vi "bats.parser.vi"(8 "FIFO In":refnum<k21>="TS-OrderBook.Command", 9 "reset":bool, 10 "data_valid":bool, 11 "data":u8) -> (3 "Ready for Input":bool)   [LabVIEW 2020]
uses:
  bats.parser.state.data.ctl
  bats.parser.state.command.ctl
  orderbook/orderbook.command.data.ctl
  orderbook/orderbook.command.type.ctl
  <vilib>/rvi/DataTransferAndStorage/Container/Common/niFpgaContainerExecOnDevCompGetState.vi
  <vilib>/rvi/Emulation/niFpgaEmulationIsFPGAContextNoSignature.vi
  <vilib>/rvi/Emulation/niFpgaSctlEmulationGetInTimedLoop.vi
  <vilib>/rvi/errors/niFpgaSetErrorForExecOnDevCompSimple.vi
  <vilib>/rvi/eio/common/nirviEmuReportErrorAndStop.vi
  <vilib>/rvi/DataTransferAndStorage/Container/Common/niFpgaContainerGetUniqueNameForEmu.vi
  <vilib>/rvi/FIFO/Fifo_Resource/nirvififoEmulationSetSize.vi
  <vilib>/rvi/FIFO/Fifo_Resource/nirviFifoEmulationQueueMgr.vi
  <instcachedir>/0/nirviFifoEmulationQueueMgr_E5CAEC123FF24DC58D834DCA3CDAA9B5.lvgen/nirviFifoEmulationQueueMgr_E5CAEC123FF24DC58D834DCA3CDAA9B5_016.vi
  <vilib>/rvi/FIFO/Fifo_Resource/nirvififoEmulationDetermineInputValidOut.vi
  <vilib>/rvi/FIFO/Fifo_Resource/nirvififoEmulationCreateLock.vi
  <vilib>/rvi/Emulation/niFpgaProcessEmulError.vi
  <vilib>/rvi/FIFO/Fifo_Resource/nirvififoEmulationObtainLock.vi
  <vilib>/rvi/FIFO/Fifo_Resource/nirvififoEmulationReleaseLock.vi
  <vilib>/rvi/occurrence/nirviWaitOnOccurrenceBase.vi
  <vilib>/rvi/errors/nirviReportUnexpectedCaseInternalError.vi
  <vilib>/rvi/errors/nirviReportUnexpectedCaseInternalError (U32).vi
  <vilib>/Utility/error.llb/Clear Errors.vi
  <vilib>/rvi/interface/RandomDataEmulation/niFpgaRandomDataHandleErrors.vi
  <vilib>/rvi/DataTransferAndStorage/Container/XNode/niFpgaContainer.xnode
  <vilib>/rvi/FIFO/Fifo_Resource/niFpgaFifoEmulationRefIn.vi
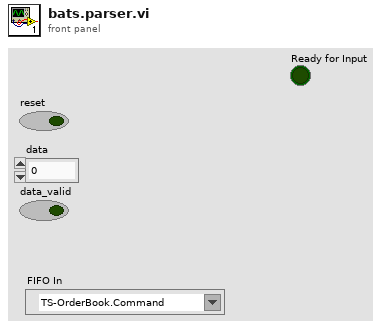
[diagram p1: front panel]
types:
  T1 = typedef "bats.parser.state.command.ctl" = enum16{"Send.Command", "Reset", "No.Op", "Read.Sequenced.Unit.Header", "Read.Msg.Type.and.Length", "Read.Time", "Read.Add.Order", "Read.Order.Executed", "Read.Reduce.Size", "Read.Modify.Order", "Read.Delete.Order"}
  T2 = typedef "orderbook.command.data.ctl" = cluster{"OrderBook Command":T3, "Side (U8)":u8, "Order Id (U64)":u64, "Quantity (U32)":u32, "Symbol (U64)":u64, "Price (U64)":u64, "Executed Quantity (U32)":u32, "Cancelled Quantity (U32)":u32}
  T3 = typedef "orderbook.command.type.ctl" = enum16{"AddOrder", "OrderExecuted", "ReduceSize", "ModifyOrder", "DeleteOrder"}
  T4 = typedef "bats.parser.state.data.ctl" = cluster{"BATS.Parser.States":T1, "Hdr Length (U16)":u16, "MessageLength (U8)":u8, "MessageType (U8)":u8, "Time (U32)":u32, "Total Counter (U16)":u16, "Message Counter (U8)":u8}
  T5 = cluster{"BATS.Parser.States":enum16{"Read.Sequenced.Unit.Header", "Read.Msg.Type.and.Length", "Read.Time", "Read.Add.Order", "Read.Order.Executed", "Read.Reduce.Size", "Read.Modify.Order", "Read.Delete.Order"}, "Hdr Length (U16)":u16, "MessageLength (U8)":u8, "MessageType (U8)":u8, "Time (U32)":u32, "Total Counter (U16)":u16, "Message Counter (U8)":u8}
  T6 = cluster{"OrderBook Command":enum16{"AddOrder", "OrderExecuted", "ReduceSize", "ModifyOrder", "DeleteOrder"}, "Side (U8)":u8, "Order Id (U64)":u64, "Quantity (U32)":u32, "Symbol (U64)":u64, "Price (U64)":u64, "Executed Quantity (U32)":u32, "Cancelled Quantity (U32)":u32}
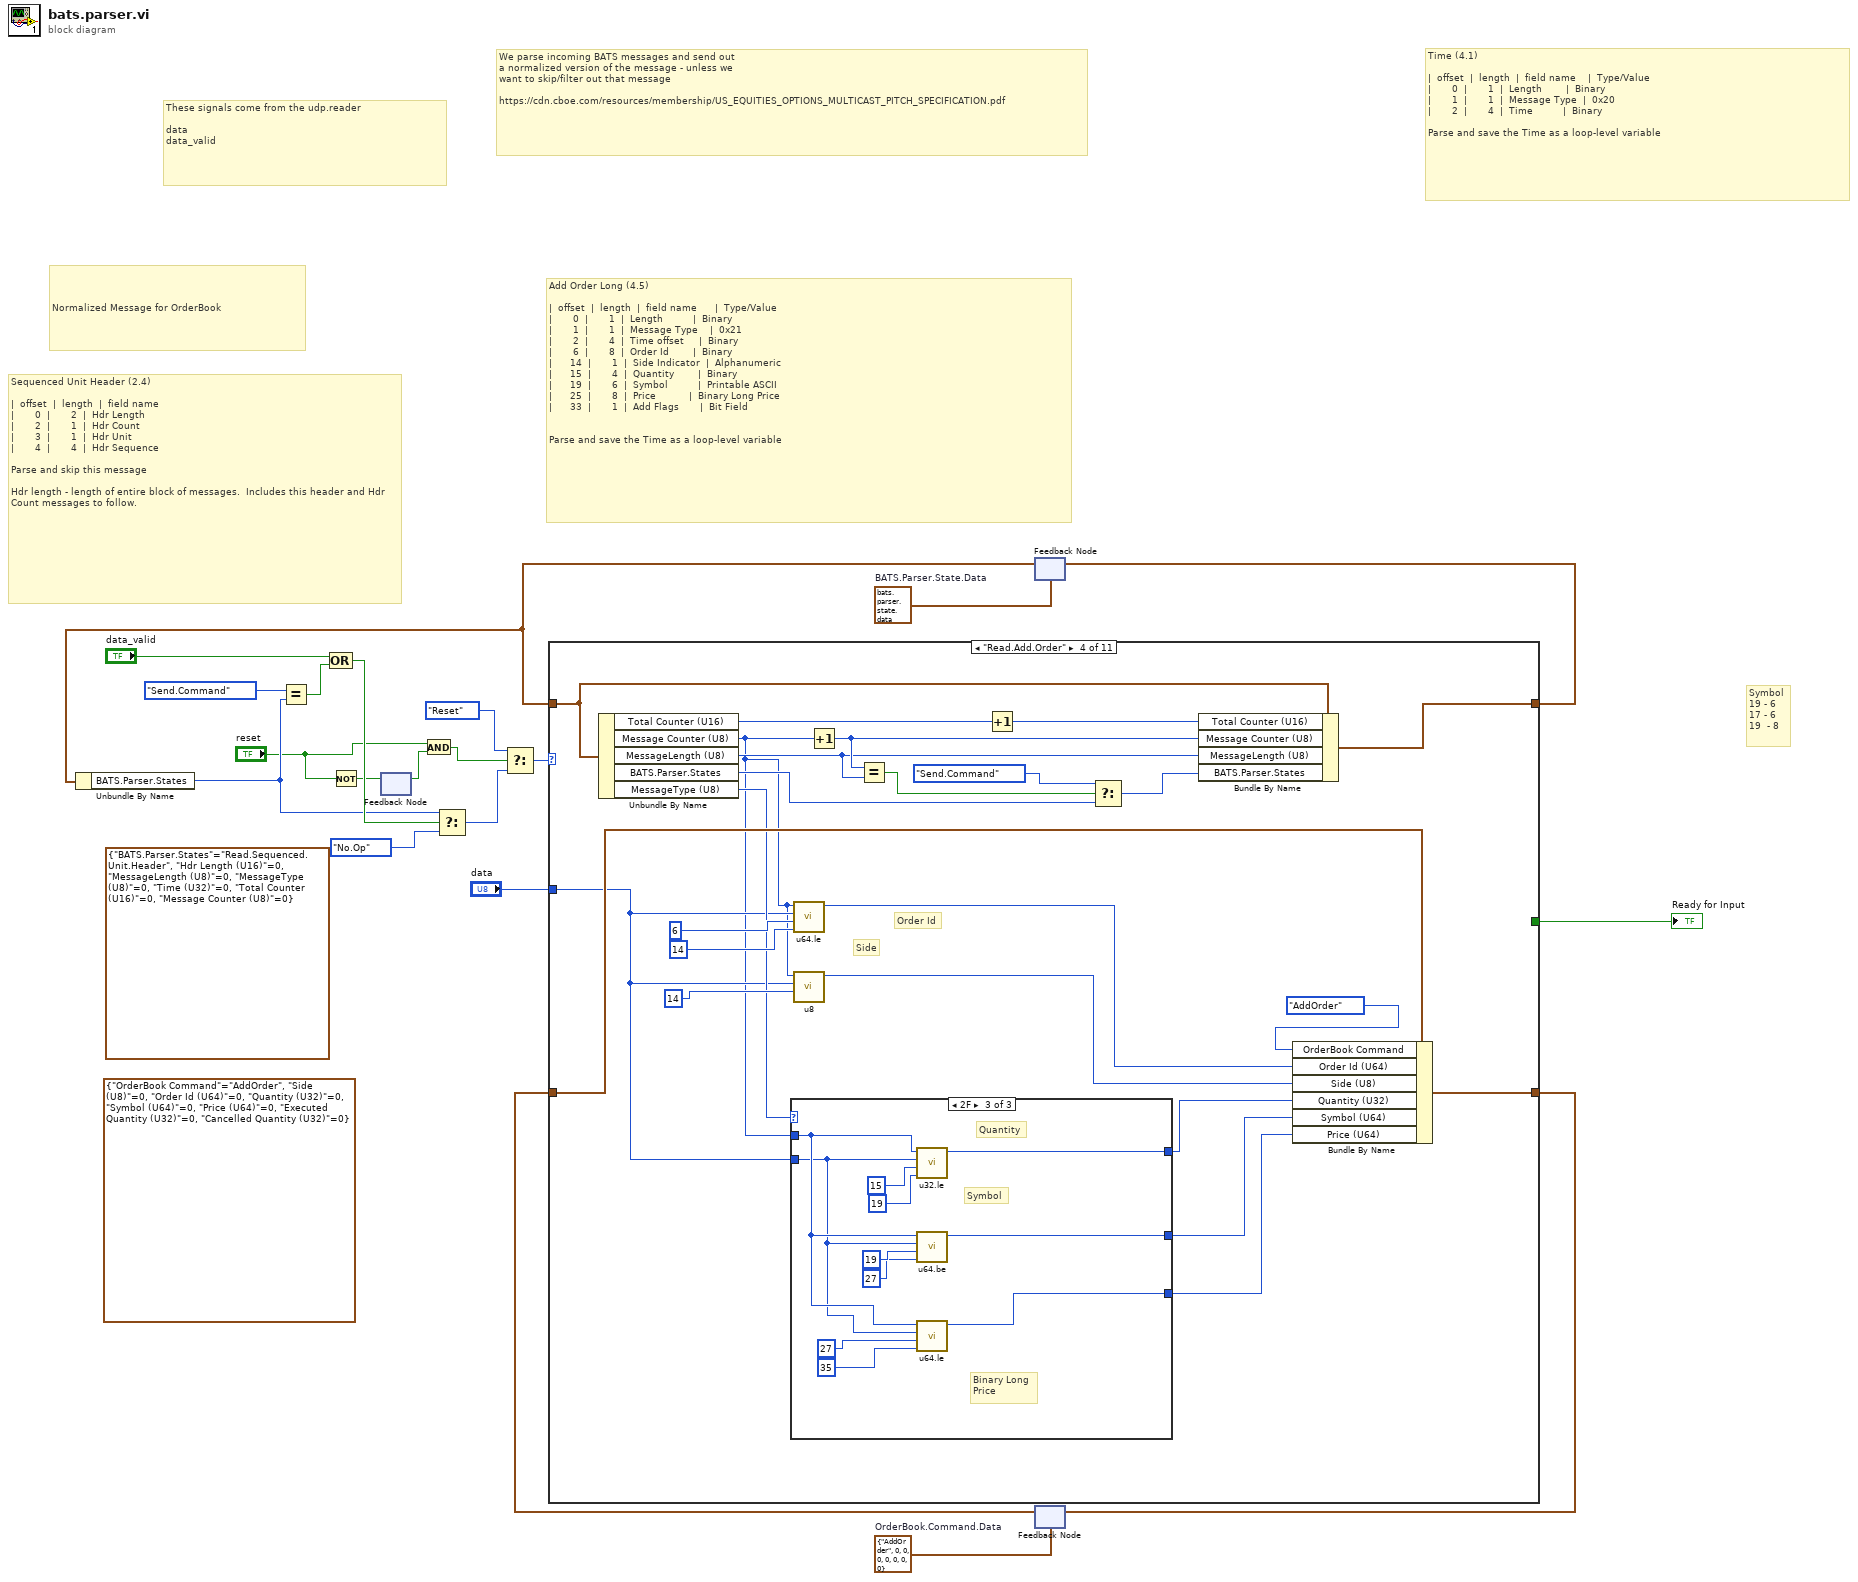
[diagram p0: block diagram]
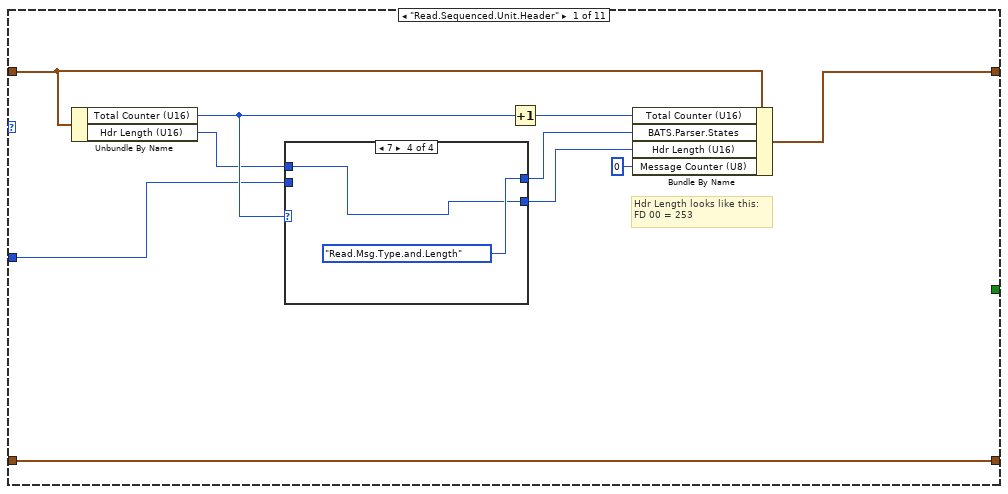
[diagram p2: hidden frame]
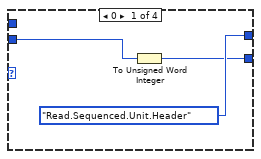
[diagram p3: hidden frame]
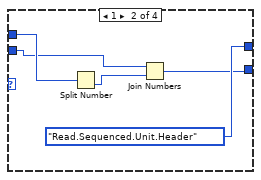
[diagram p4: hidden frame]
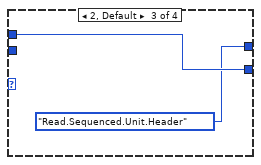
[diagram p5: hidden frame]
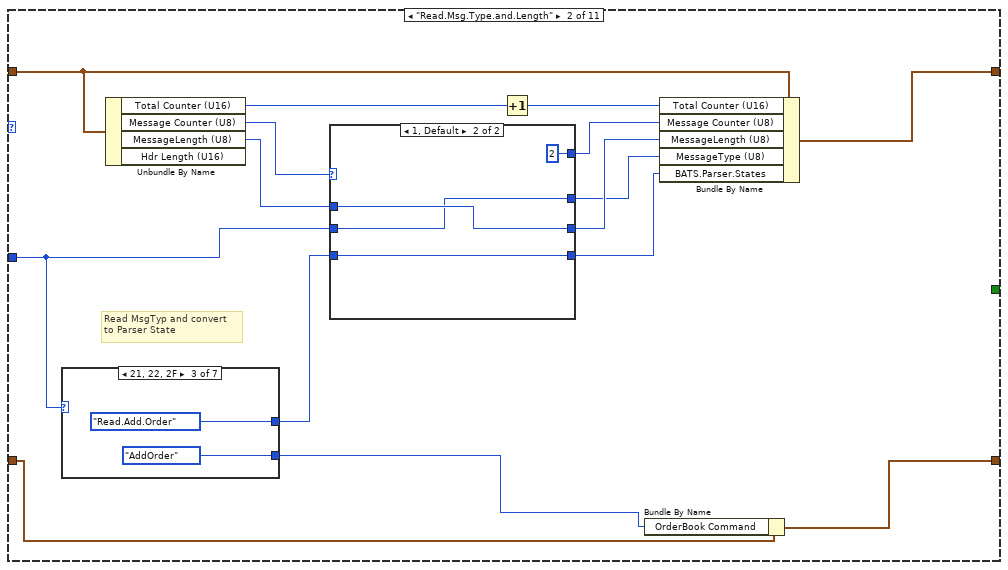
[diagram p6: hidden frame]
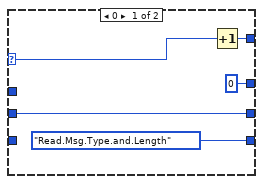
[diagram p7: hidden frame]
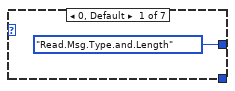
[diagram p8: hidden frame]
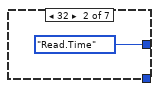
[diagram p9: hidden frame]
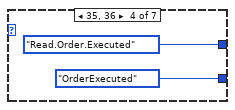
[diagram p10: hidden frame]
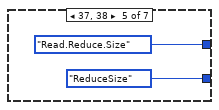
[diagram p11: hidden frame]
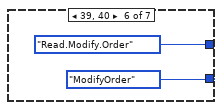
[diagram p12: hidden frame]
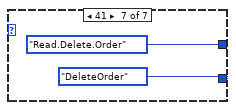
[diagram p13: hidden frame]
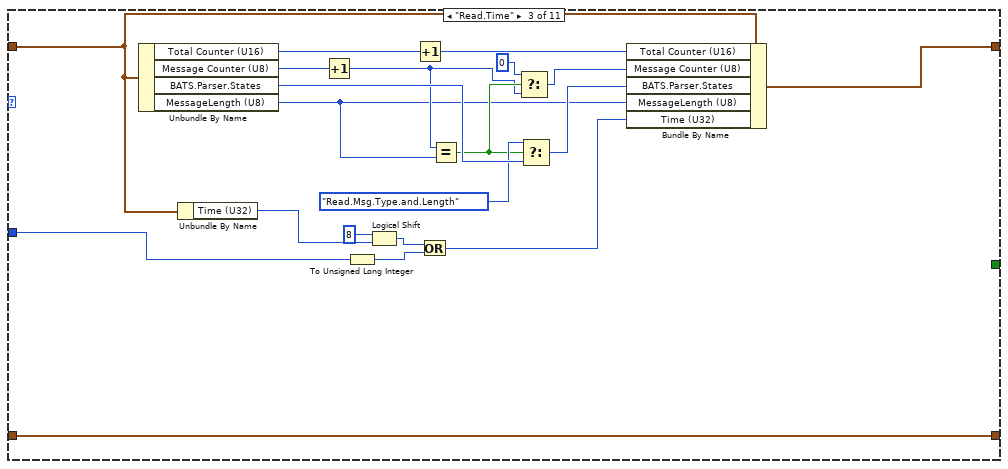
[diagram p14: hidden frame]
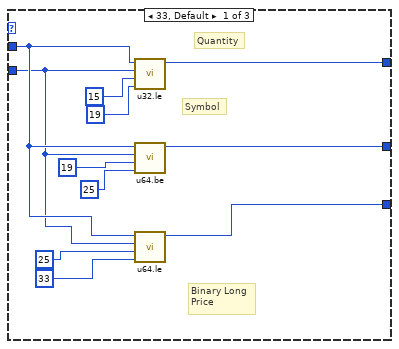
[diagram p15: hidden frame]
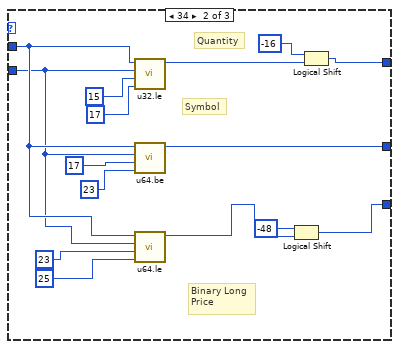
[diagram p16: hidden frame]
diagram:
  w17 = T2 {"OrderBook Command"=enum."AddOrder", "Side (U8)"=0, "Order Id (U64)"=0, "Quantity (U32)"=0, "Symbol (U64)"=0, "Price (U64)"=0, "Executed Quantity (U32)"=0, "Cancelled Quantity (U32)"=0}  # OrderBook.Command.Data
  w18 = T4 {"BATS.Parser.States"=enum."Read.Sequenced.Unit.Header", "Hdr Length (U16)"=0, "MessageLength (U8)"=0, "MessageType (U8)"=0, "Time (U32)"=0, "Total Counter (U16)"=0, "Message Counter (U8)"=0}  # BATS.Parser.State.Data
  (unwired) T5 {"BATS.Parser.States"=enum."Read.Sequenced.Unit.Header", "Hdr Length (U16)"=0, "MessageLength (U8)"=0, "MessageType (U8)"=0, "Time (U32)"=0, "Total Counter (U16)"=0, "Message Counter (U8)"=0}
  (unwired) T6 {"OrderBook Command"=enum."AddOrder", "Side (U8)"=0, "Order Id (U64)"=0, "Quantity (U32)"=0, "Symbol (U64)"=0, "Price (U64)"=0, "Executed Quantity (U32)"=0, "Cancelled Quantity (U32)"=0}
  # "Symbol\n19 - 6\n17 - 6\n19  - 8"
  # "Sequenced Unit Header (2.4)\n\n|  offset  |  length  |  field name\n|       0  |       2  |  Hdr Length\n|       2  |       1  |  Hdr Count\n|       3  |       1  |  Hdr Unit\n|       4  |       4  |  Hdr Sequence\n\nParse and skip this message\n\nHdr length - length of entire block of messages.  Includes this header and Hdr Count messages to follow."
  # "Normalized Message for OrderBook"
  # "Add Order Long (4.5)\n\n|  offset  |  length  |  field name      |  Type/Value\n|       0  |       1  |  Length          |  Binary\n|       1  |       1  |  Message Type    |  0x21\n|       2  |       4  |  Time offset     |  Binary\n|       6  |       8  |  Order Id        |  Binary\n|      14  |       1  |  Side Indicator  |  Alphanumeric\n|      15  |       4  |  Quantity        |  Binary\n|      19  |       6  |  Symbol          |  Printable ASCII\n|      25  |       8  |  Price           |  Binary Long Price\n|      33  |       1  |  Add Flags       |  Bit Field\n\n\nParse and save the Time as a loop-level variable"
  # "Time (4.1)\n\n|  offset  |  length  |  field name    |  Type/Value\n|       0  |       1  |  Length        |  Binary\n|       1  |       1  |  Message Type  |  0x20\n|       2  |       4  |  Time          |  Binary\n\nParse and save the Time as a loop-level variable"
  # "We parse incoming BATS messages and send out\na normalized version of the message - unless we\nwant to skip/filter out that message\n\nhttps://cdn.cboe.com/resources/membership/US_EQUITIES_OPTIONS_MULTICAST_PITCH_SPECIFICATION.pdf"
  # "These signals come from the udp.reader\n\ndata\ndata_valid"
  n1 = Not(x="reset") -> (.not. x?=w2:bool)
  n2 = feedback-in #1(w2) -> ()
  n3 = feedback #1() -> (w3:bool)  [unwired: 1 in]
  n4 = And(x="reset", y=w3) -> (x .and. y?=w4:bool)
  n5 = feedback #2(w18) -> (w14:T4)
  n6 = Unbundle By Name(w14) -> ("BATS.Parser.States"=w6:T1)
  n7 = Equal?(x=bats.parser.state.command."Send.Command" ("BATS.Parser.States"), y=w6) -> (x = y?=w7:bool)
  n8 = Compound Arithmetic op=OR("data_valid", w7) -> (w9:bool)
  n9 = Select(t=w6, s=w9, f=bats.parser.state.command."No.Op" ("BATS.Parser.States")) -> (s? t:f=w11:T1)
  n10 = Select(t=bats.parser.state.command."Reset" ("BATS.Parser.States"), s=w4, f=w11) -> (s? t:f=w12:T1)
  n11 = feedback #3(w17) -> (w20:T2)
  n12 = case shown="\"Read.Add.Order\"" w12 {
    tunnel: w14 -> [w27 w57 w90 w119 w161 w163 w165 w167 _ w190 w200]
    tunnel: [w25 w54 w84 w116 w162 w164 w166 w168 w174 w189 w194] -> w21
    tunnel: w20 -> [w25 w55 w84 w114 w162 w164 w166 w168 _ w189 w194]
    tunnel: [w30 w58 w98 w117 w161 w163 w165 w167 w186 w190 w199] -> w19
    tunnel: "data" -> [w23 w47 w80 w102 _ _ _ _ _ _ _]
    tunnel: [_ _ _ _ _ _ _ _ _ TRUE ("Ready for Input") w191] -> w1
    frame "Read.Sequenced.Unit.Header" {
      # "Hdr Length looks like this:\nFD 00 = 253"
      n13 = Unbundle By Name(w27) -> ("Total Counter (U16)"=w29:u16, "Hdr Length (U16)"=w28:u16)
      n14 = case shown="7" w29 {
        tunnel: w28 -> [_ w38 w41 w42]
        tunnel: w23 -> [w33 w37 _ _]
        tunnel: [w32 w35 w41 w42] -> w22
        tunnel: [bats.parser.state.command."Read.Sequenced.Unit.Header" ("BATS.Parser.States") bats.parser.state.command."Read.Sequenced.Unit.Header" ("BATS.Parser.States") bats.parser.state.command."Read.Sequenced.Unit.Header" ("BATS.Parser.States") bats.parser.state.command."Read.Msg.Type.and.Length" ("BATS.Parser.States")] -> w26
        frame 0 {
          n15 = To Unsigned Word Integer(number=w33) -> (unsigned 16bit integer=w32:u16)
        }
        frame 1 {
          n16 = Split Number(x=w38) -> (lo(x)=w36:u8)  [unwired: 1 out]
          n17 = Join Numbers(hi=w37, lo=w36) -> ((hi.lo)=w35:u16)
        }
        frame 2, Default {
        }
        frame 7 {
        }
      }
      n18 = Increment(x=w29) -> (x+1=w24:u16)
      n19 = Bundle By Name(cluster=w27, "Total Counter (U16)"=w24, "BATS.Parser.States"=w26, "Hdr Length (U16)"=w22, "Message Counter (U8)"=u8 0) -> (w30:T4)
    }
    frame "Read.Msg.Type.and.Length" {
      # "Read MsgTyp and convert\nto Parser State"
      n20 = case shown="21, 22, 2F" w47 {
        tunnel: [bats.parser.state.command."Read.Msg.Type.and.Length" ("BATS.Parser.States") bats.parser.state.command."Read.Time" ("BATS.Parser.States") bats.parser.state.command."Read.Add.Order" ("BATS.Parser.States") bats.parser.state.command."Read.Order.Executed" ("BATS.Parser.States") bats.parser.state.command."Read.Reduce.Size" ("BATS.Parser.States") bats.parser.state.command."Read.Modify.Order" ("BATS.Parser.States") bats.parser.state.command."Read.Delete.Order" ("BATS.Parser.States")] -> w49
        tunnel: [_ _ orderbook.command.type."AddOrder" ("OrderBook Command") orderbook.command.type."OrderExecuted" ("OrderBook Command") orderbook.command.type."ReduceSize" ("OrderBook Command") orderbook.command.type."ModifyOrder" ("OrderBook Command") orderbook.command.type."DeleteOrder" ("OrderBook Command")] -> w53
        frame 0, Default {
        }
        frame 32 {
        }
        frame 33, 34, 47 {
        }
        frame 35, 36 {
        }
        frame 37, 38 {
        }
        frame 39, 40 {
        }
        frame 41 {
        }
      }
      n21 = Unbundle By Name(w57) -> ("Total Counter (U16)"=w45:u16, "Message Counter (U8)"=w46:u8, "MessageLength (U8)"=w52:u8)  [unwired: 1 out]
      n22 = case shown="1, Default" w46 {
        selector: w46 -> [w60 _]
        tunnel: w52 -> [_ w67]
        tunnel: [w63 w67] -> w51
        tunnel: w47 -> [w63 w66]
        tunnel: [bats.parser.state.command."Read.Msg.Type.and.Length" ("BATS.Parser.States") w65] -> w50
        tunnel: w49 -> [_ w65]
        tunnel: [u8 0 ("data") w66] -> w48
        tunnel: [w59 u8 2] -> w44
        frame 0 {
          n23 = Increment(x=w60) -> (x+1=w59:u8)
        }
        frame 1, Default {
        }
      }
      n24 = Increment(x=w45) -> (x+1=w56:u16)
      n25 = Bundle By Name(cluster=w55, "OrderBook Command"=w53) -> (w54:T2)
      n26 = Bundle By Name(cluster=w57, "Total Counter (U16)"=w56, "Message Counter (U8)"=w44, "MessageLength (U8)"=w51, "MessageType (U8)"=w48, "BATS.Parser.States"=w50) -> (w58:T4)
    }
    frame "Read.Time" {
      n27 = Unbundle By Name(w90) -> ("Total Counter (U16)"=w99:u16, "Message Counter (U8)"=w81:u8, "BATS.Parser.States"=w96:T1, "MessageLength (U8)"=w82:u8)
      n28 = Unbundle By Name(w90) -> ("Time (U32)"=w89:u32)
      n29 = Increment(x=w81) -> (x+1=w83:u8)
      n30 = To Unsigned Long Integer(number=w80) -> (unsigned 32bit integer=w91:u32)
      n31 = Logical Shift(y=i16 8, x=w89) -> (x << y=w92:u32)
      n32 = Increment(x=w99) -> (x+1=w97:u16)
      n33 = Or(x=w92, y=w91) -> (x .or. y?=w88:u32)
      n34 = Equal?(x=w83, y=w82) -> (x = y?=w86:bool)
      n35 = Select(t=u8 0, s=w86, f=w83) -> (s? t:f=w87:u8)
      n36 = Select(t=bats.parser.state.command."Read.Msg.Type.and.Length", s=w86, f=w96) -> (s? t:f=w94:T1)
      n37 = Bundle By Name(cluster=w90, "Total Counter (U16)"=w97, "Message Counter (U8)"=w87, "BATS.Parser.States"=w94, "MessageLength (U8)"=w82, "Time (U32)"=w88) -> (w98:T4)
    }
    frame "Read.Add.Order" {
      # "Side"
      # "Order Id"
      n38 = Unbundle By Name(w119) -> ("Total Counter (U16)"=w123:u16, "Message Counter (U8)"=w100:u8, "MessageLength (U8)"=w115:u8, "BATS.Parser.States"=w113:T1, "MessageType (U8)"=w105:u8)
      n39 = case shown="2F" w105 {
        tunnel: w102 -> [w126 w143 w152]
        tunnel: w100 -> [w127 w144 w153]
        tunnel: [w132 w138 w158] -> w104
        tunnel: [w131 w147 w157] -> w103
        tunnel: [w128 w136 w154] -> w101
        frame 33, Default {
          # "Binary Long\nPrice"
          # "Symbol"
          # "Quantity"
          n40 = call "u32.le.vi"("end"=u8 19, "start"=u8 15, "Data"=w126, "Counter"=w127) -> ("Latched\nValue"=w132:u32)  [unwired: 7 in]
          n41 = call "u64.be.vi"("end"=u8 25, "start"=u8 19, "Data"=w126, "Counter"=w127) -> ("Latched\nValue"=w131:u64)  [unwired: 7 in]
          n42 = call "u64.le.vi"("end"=u8 33, "start"=u8 25, "Data"=w126, "Counter"=w127) -> ("Latched\nValue"=w128:u64)  [unwired: 7 in]
        }
        frame 34 {
          # "Binary Long\nPrice"
          # "Symbol"
          # "Quantity"
          n43 = call "u32.le.vi"("end"=u8 17, "start"=u8 15, "Data"=w143, "Counter"=w144) -> ("Latched\nValue"=w140:u32)  [unwired: 7 in]
          n44 = call "u64.be.vi"("end"=u8 23, "start"=u8 17, "Data"=w143, "Counter"=w144) -> ("Latched\nValue"=w147:u64)  [unwired: 7 in]
          n45 = call "u64.le.vi"("end"=u8 25, "start"=u8 23, "Data"=w143, "Counter"=w144) -> ("Latched\nValue"=w137:u64)  [unwired: 7 in]
          n46 = Logical Shift(y=i16 -48, x=w137) -> (x << y=w136:u64)
          n47 = Logical Shift(y=i16 -16, x=w140) -> (x << y=w138:u32)
        }
        frame 47 {
          # "Binary Long\nPrice"
          # "Symbol"
          # "Quantity"
          n48 = call "u32.le.vi"("end"=u8 19, "start"=u8 15, "Data"=w152, "Counter"=w153) -> ("Latched\nValue"=w158:u32)  [unwired: 7 in]
          n49 = call "u64.be.vi"("end"=u8 27, "start"=u8 19, "Data"=w152, "Counter"=w153) -> ("Latched\nValue"=w157:u64)  [unwired: 7 in]
          n50 = call "u64.le.vi"("end"=u8 35, "start"=u8 27, "Data"=w152, "Counter"=w153) -> ("Latched\nValue"=w154:u64)  [unwired: 7 in]
        }
      }
      n51 = call "u64.le.vi"("end"=u8 14, "start"=u8 6, "Data"=w102, "Counter"=w100) -> ("Latched\nValue"=w106:u64)  [unwired: 7 in]
      n52 = call "u8.vi"("idx"=u8 14 ("x"), "data in"=w102, "Message Counter (U8)"=w100) -> ("data out"=w107:u8)  [unwired: 8 in]
      n53 = Increment(x=w100) -> (x+1=w121:u8)
      n54 = Equal?(x=w121, y=w115) -> (x = y?=w120:bool)
      n55 = Increment(x=w123) -> (x+1=w122:u16)
      n56 = Select(t=bats.parser.state.command."Send.Command" ("BATS.Parser.States"), s=w120, f=w113) -> (s? t:f=w112:T1)
      n57 = Bundle By Name(cluster=w119, "Total Counter (U16)"=w122, "Message Counter (U8)"=w121, "MessageLength (U8)"=w115, "BATS.Parser.States"=w112) -> (w117:T4)
      n58 = Bundle By Name(cluster=w114, "OrderBook Command"=orderbook.command.type."AddOrder", "Order Id (U64)"=w106, "Side (U8)"=w107, "Quantity (U32)"=w104, "Symbol (U64)"=w103, "Price (U64)"=w101) -> (w116:T2)
    }
    frame "Read.Order.Executed" {
    }
    frame "Read.Reduce.Size" {
    }
    frame "Read.Modify.Order" {
    }
    frame "Read.Delete.Order" {
    }
    frame "Reset" {
      w183 = T2 {"OrderBook Command"=enum."AddOrder", "Side (U8)"=0, "Order Id (U64)"=0, "Quantity (U32)"=0, "Symbol (U64)"=0, "Price (U64)"=0, "Executed Quantity (U32)"=0, "Cancelled Quantity (U32)"=0}  # OrderBook.Command.Data
      w187 = T4 {"BATS.Parser.States"=enum."Read.Sequenced.Unit.Header", "Hdr Length (U16)"=0, "MessageLength (U8)"=0, "MessageType (U8)"=0, "Time (U32)"=0, "Total Counter (U16)"=0, "Message Counter (U8)"=0}  # BATS.Parser.States
      n59 = Bundle By Name(cluster=w187, "BATS.Parser.States"=bats.parser.state.command."Read.Sequenced.Unit.Header", "Hdr Length (U16)"=u16 0, "MessageLength (U8)"=u8 0, "MessageType (U8)"=u8 0, "Time (U32)"=u32 0, "Total Counter (U16)"=u16 0, "Message Counter (U8)"=u8 0) -> (w186:T4)
      n60 = Bundle By Name(cluster=w183, "OrderBook Command"=orderbook.command.type."AddOrder", "Side (U8)"=u8 0, "Order Id (U64)"=u64 0, "Quantity (U32)"=u32 0, "Symbol (U64)"=u64 11111, "Price (U64)"=u64 0, "Executed Quantity (U32)"=u32 0, "Cancelled Quantity (U32)"=u32 0) -> (w174:T2)
    }
    frame "No.Op", Default {
    }
    frame "Send.Command" {
      n61 = Unbundle By Name(w200) -> ("BATS.Parser.States"=w196:T1)
      n62 = feedback #4(FALSE ("Ready for Input")) -> (w191:bool)
      n63 = Select(t=bats.parser.state.command."Read.Msg.Type.and.Length" ("BATS.Parser.States"), s=w191, f=w196) -> (s? t:f=w197:T1)
      n64 = xnode "FIFO Write Using Handshaking"("Element"=w194, "Input Valid"=w191, "FIFO In"="FIFO In") -> ("Ready for Input"=w192:bool)  [unwired: 1 out]
      n65 = feedback-in #4(w192) -> ()
      n66 = Bundle By Name(cluster=w200, "BATS.Parser.States"=w197, "Message Counter (U8)"=u8 0) -> (w199:T4)
    }
  }
  "Ready for Input" <- w1
  n67 = feedback-in #2(w19) -> ()
  n68 = feedback-in #3(w21) -> ()
